vi "Write Controller Actor Enqueuer.vi"(8 "error in (no error)":errorcluster, 10 "Controller Actor Enqueuer":refnum<class "Message Enqueuer.lvclass">, 11 "View in":refnum<class "View.lvclass">) -> (0 "error out":errorcluster, 3 "View out":refnum<class "View.lvclass">)   [LabVIEW 2023, in "MVC Actors.lvlib" / "View.lvclass"]
uses:
  View.lvclass
  <vilib>/ActorFramework/Message Enqueuer/Message Enqueuer.lvclass
  View.lvclass/View.ctl
  Controller Messages/Finalize View Init Msg/Finalize View Init Msg.lvclass
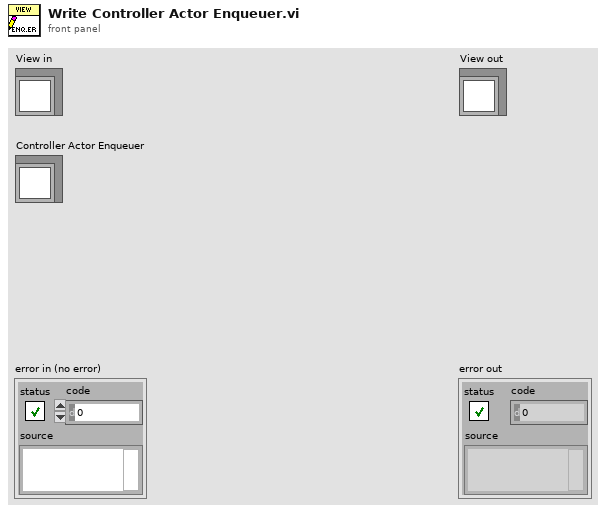
[diagram p1: front panel]
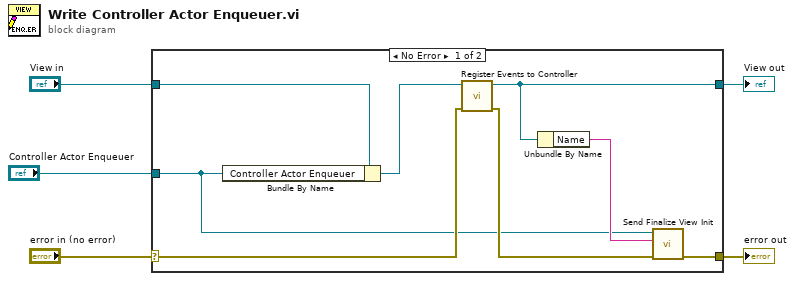
[diagram p0: block diagram]
diagram:
  n1 = case shown="No Error" "error in (no error)" {
    selector: "error in (no error)" -> [w11 w14]
    tunnel: [w9 w14] -> w4
    tunnel: [w8 w15] -> w2
    tunnel: "View in" -> [w13 w15]
    tunnel: "Controller Actor Enqueuer" -> [w6 _]
    frame No Error {
      n2 = Bundle By Name(cluster=w13, "Controller Actor Enqueuer"=w6) -> (w12:refnum<class "View.lvclass">)
      n3 = call-dynamic "Register Events to Controller.vi"("error in (no error)"=w11, "View Actor in"=w12) -> ("error out"=w10:errorcluster, "View Actor out"=w8:refnum<class "View.lvclass">)  [unwired: 8 in]
      n4 = Unbundle By Name(w8) -> ("Name"=w7:string)
      n5 = call "Send Finalize View Init.vi"("error in (no error)"=w10, "View Name"=w7, "Message Enqueuer in"=w6) -> ("error out"=w9:errorcluster)  [unwired: 7 in, 1 out]
    }
    frame Error {
    }
  }
  "error out" <- w4
  "View out" <- w2
